vi "Practica11_Ethernet.vi"() -> ()   [LabVIEW 2015]
panel:
  out "String":string
  in  "stop":bool
  in  "LED":bool
  out "Potenciometro":dbl(knob) scale=0.0..1023.0
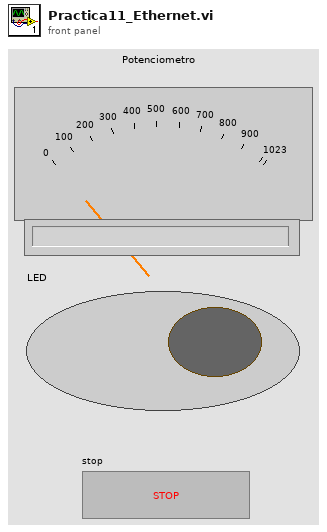
[diagram p1: front panel]
types:
  T1 = enum16{"Standard", "Buffered", "CRLF", "Immediate"}
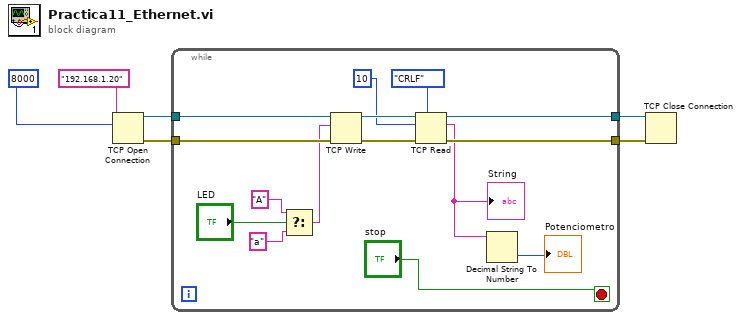
[diagram p0: block diagram]
diagram:
  n1 = TCP Open Connection(address="192.168.1.20", remote port or service name=u16 8000) -> (connection ID=w6:refnum<k5>, error out=w5:errorcluster)  [unwired: 3 in]
  n2 = while {
    tunnel: w6 -> [w21]
    tunnel: w5 -> [w20]
    tunnel: [w17] -> w2
    tunnel: [w16] -> w1
    stop <- "stop" stop-if-true
    n3 = Select(t="A", s="LED", f="a") -> (s? t:f=w12:string)
    n4 = TCP Write(connection ID=w21, data in=w12, error in (no error)=w20) -> (connection ID out=w18:refnum<k5>, error out=w19:errorcluster)  [unwired: 1 in, 1 out]
    n5 = TCP Read(connection ID=w18, bytes to read=10, error in (no error)=w19, 7:T1."CRLF" ("mode (standard)")) -> (connection ID out=w17:refnum<k5>, data out=w9:string, error out=w16:errorcluster)  [unwired: 1 in]
    "String" <- w9
    n6 = Decimal String To Number(string=w9) -> (number=→"Potenciometro":i32)  [unwired: 2 in, 1 out]
  }
  n7 = TCP Close Connection(connection ID=w2, error in (no error)=w1) -> ()  [unwired: 1 in, 2 out]
